vi "PRINT_LABEL.vi"(9 "CURRENT_YEAR_DATA":string, 10 "ECODE 2":string, 11 "connection reference":T1) -> ()   [LabVIEW 2015]
uses:
  <vilib>/addons/database/Connection.llb/Conn ObjectReference.ctl
  Controls/ITEM_INFORMATION_CLUSTER.ctl
  <vilib>/addons/database/_DB Variant To Data/Database Variant To Data.xnode
  <vilib>/addons/database/NI_Database_API.lvlib
  <vilib>/addons/database/Connection.llb/DB Tools Open Connec (String).vi
panel:
  in  "Search button":bool
  in  "Lot Maker":string
  out "Find Array":i32[](array[numeric])
  in  "Location":string
  in  "Maker Code":string
  in  "BUTTON_EXIT":bool
  in  "BUTTON_PRINT":bool
  in  "BUTTON_ADD":bool
  in  "Amount":dbl
  in  "Unit 2":string
  in  "Quantity":dbl
  in  "Lot Size":dbl
  in  "Unit":string
  in  "Item Code (F3)":string
  in  "Part No.(F2)":string
  in  "Barcode (F1)":string
  in  "Offset":dbl
  in  "Length":dbl
  in  "Maker":string(combo)
  in  "Part Name":string(combo)
  in  "Product":string(combo)
  out "ECODE":string
  in  "Invoice Date":timestamp format="%<%d/%m/%Y>T"
  in  "Invoice No.":string
  # "PRINT LABEL"
  # "X"
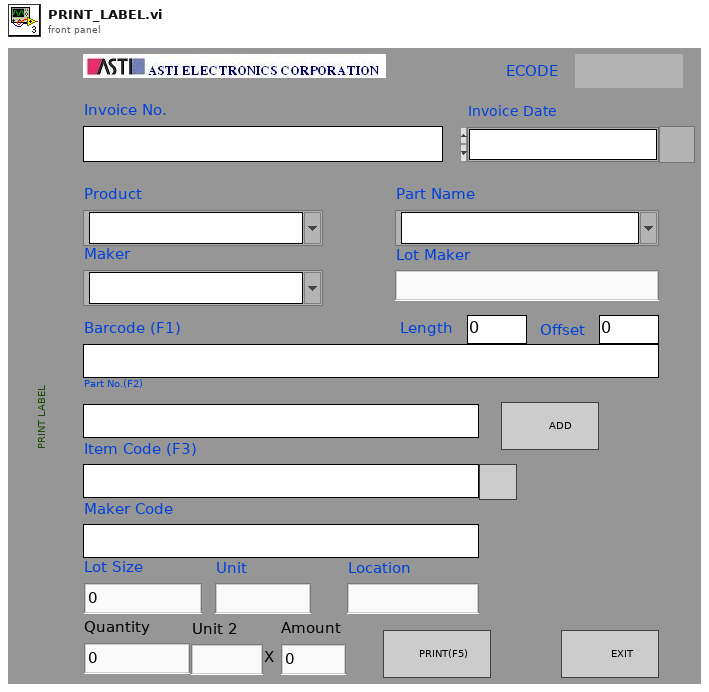
[diagram p1: front panel]
types:
  T1 = typedef "NI_Database_API.lvlib/Conn ObjectReference.ctl" = refnum<k1>
  T2 = typedef "ITEM_INFORMATION_CLUSTER.ctl" = cluster{"PRODUCT":string, "ITEM_CODE":string, "PART_NAME":string, "MAKER":string, "PART_NO":string, "LOT_SIZE":dbl, "UNIT":string, "LENGTH-OFFSET":string, "BARCODE":string, "PROCESS":string, "INVENTORY_LOCAL":string, "TARE":dbl, "SAMPLE":dbl}
  T3 = cluster{"QR_code Text":string, "Lot Maker":string, "Item Code (F3)":string, "date/time string":string, "Invoice No.":string, "Maker":string, "Part No.(F2) ":string, "Location":string, "Product":string, "Qty":string, "ECODE":string}
  T4 = cluster{"PRODUCT":string, "ITEM CODE":string, "PART NAME":string, "MAKER":string, "PART NO":string, "LOT SIZE":dbl, "UNIT":string, "LENGTH-OFFSET":string, "BARCODE":string, "PROCESS":string, "INVENTORY LOCAL":string, "TARE":dbl, "SAMPLE":dbl}
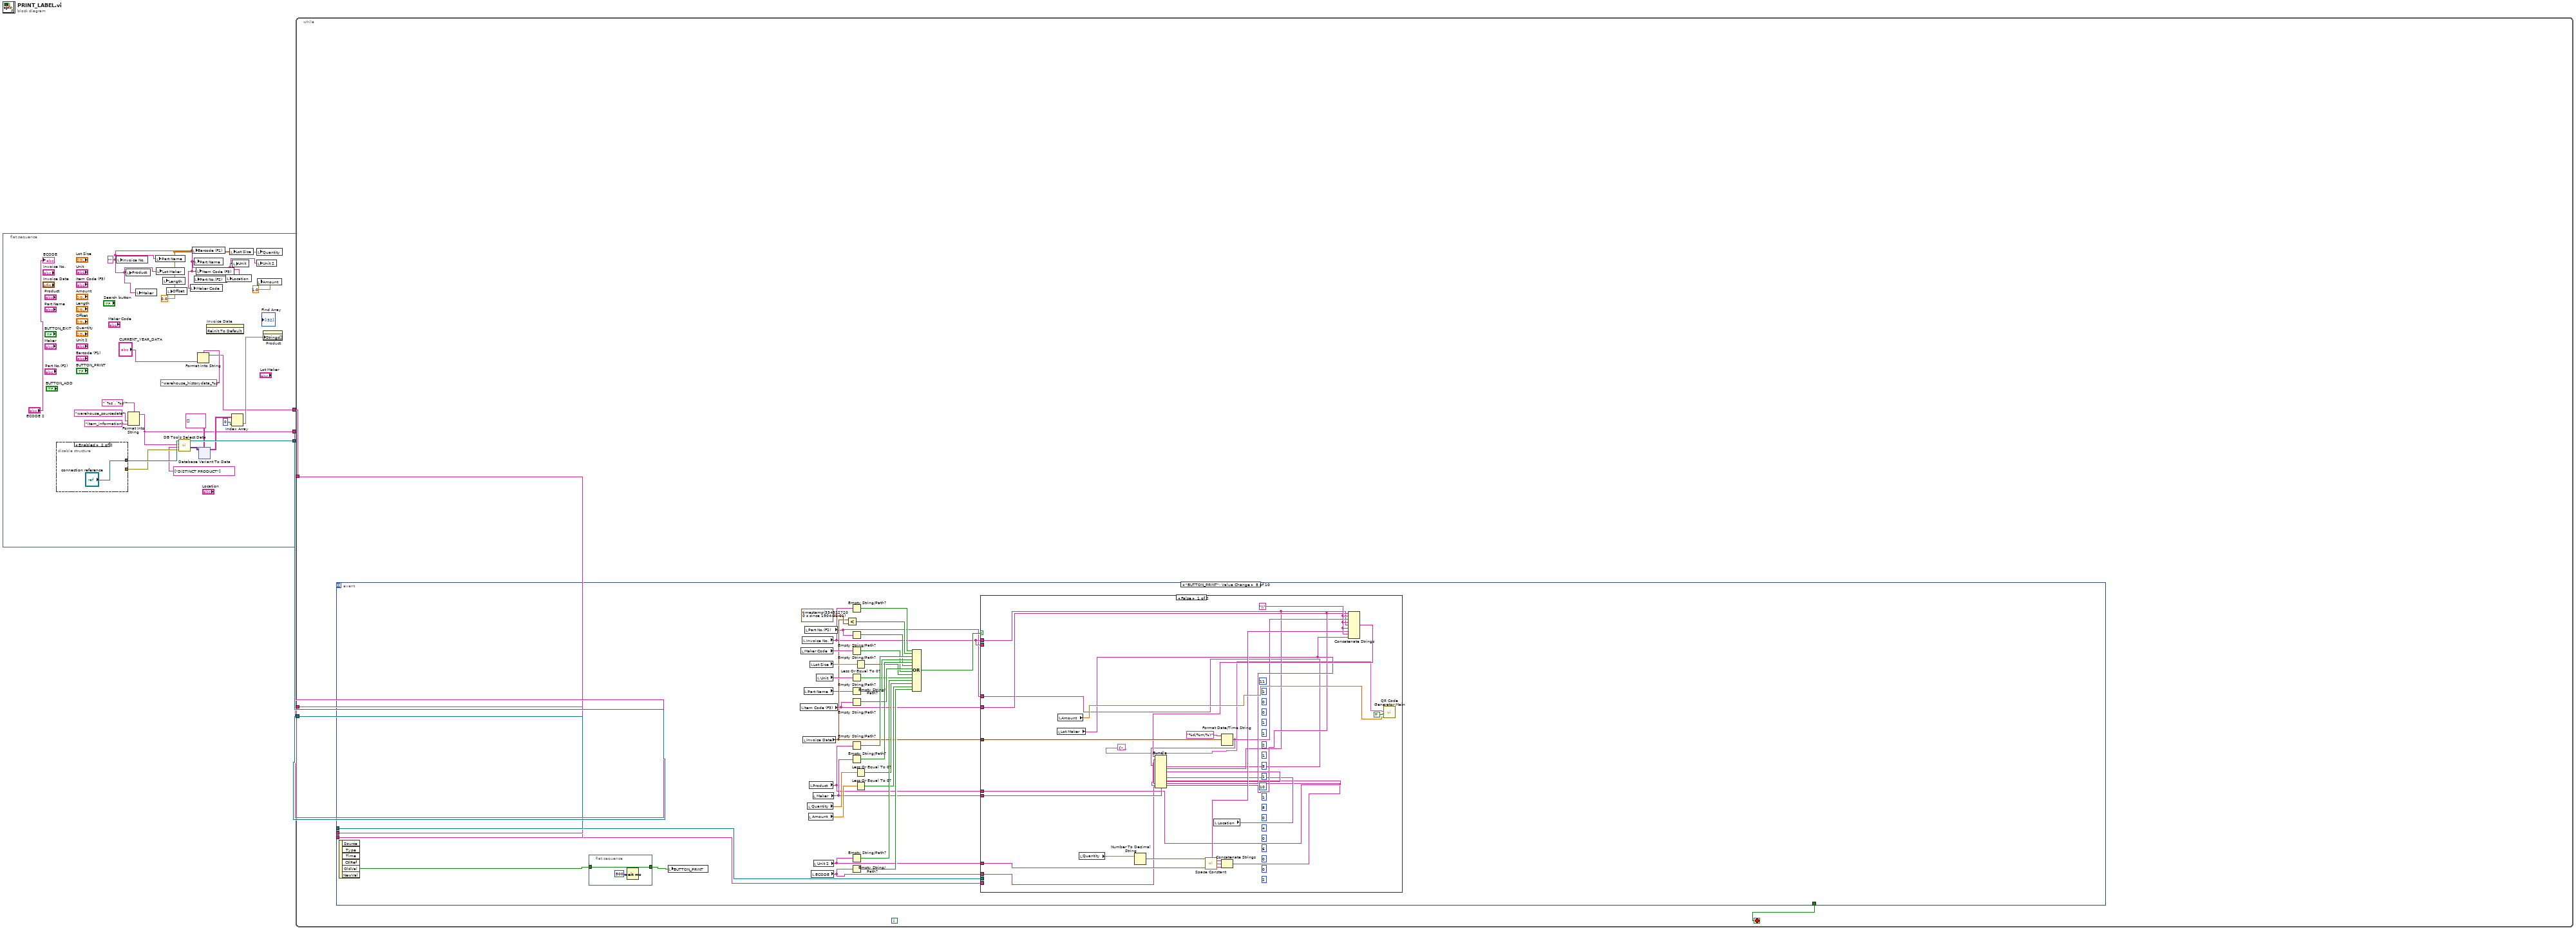
[diagram p0: block diagram]
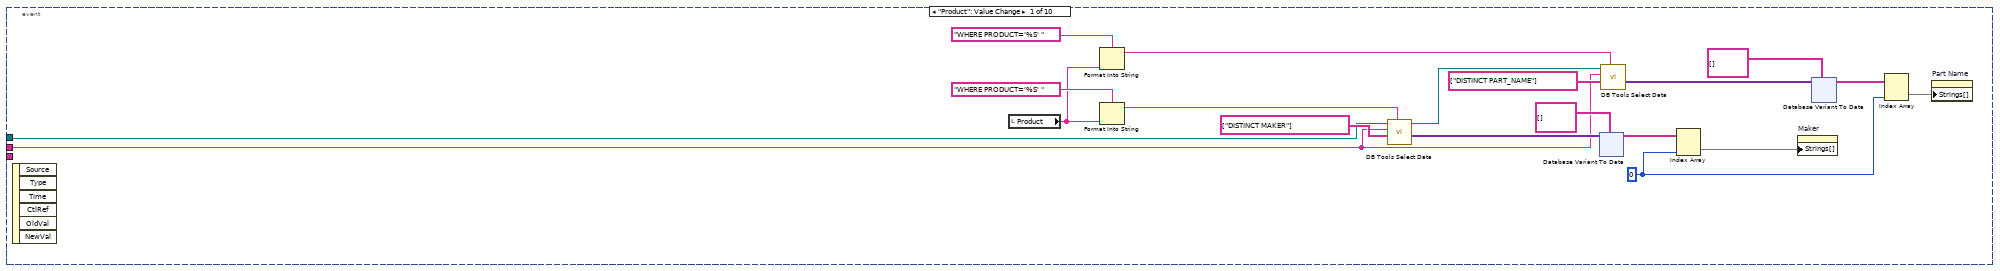
[diagram p2: hidden frame]
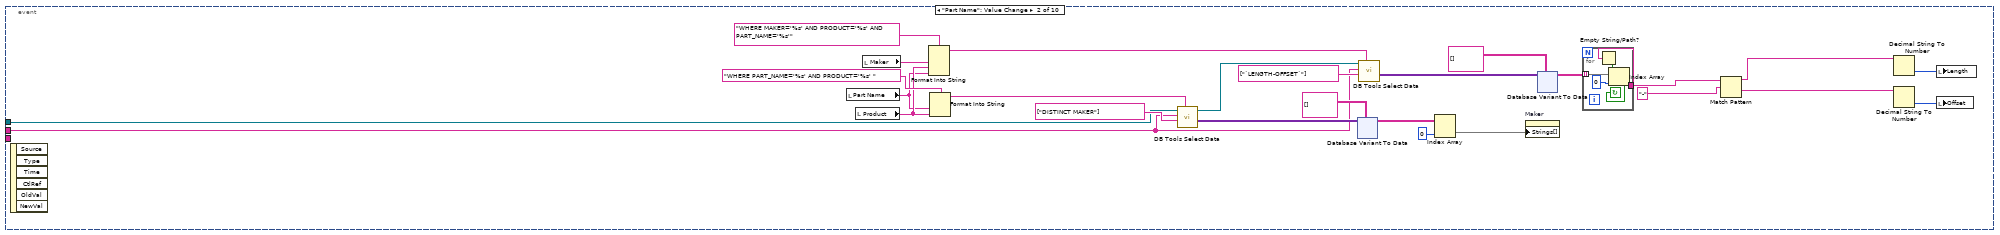
[diagram p3: hidden frame]
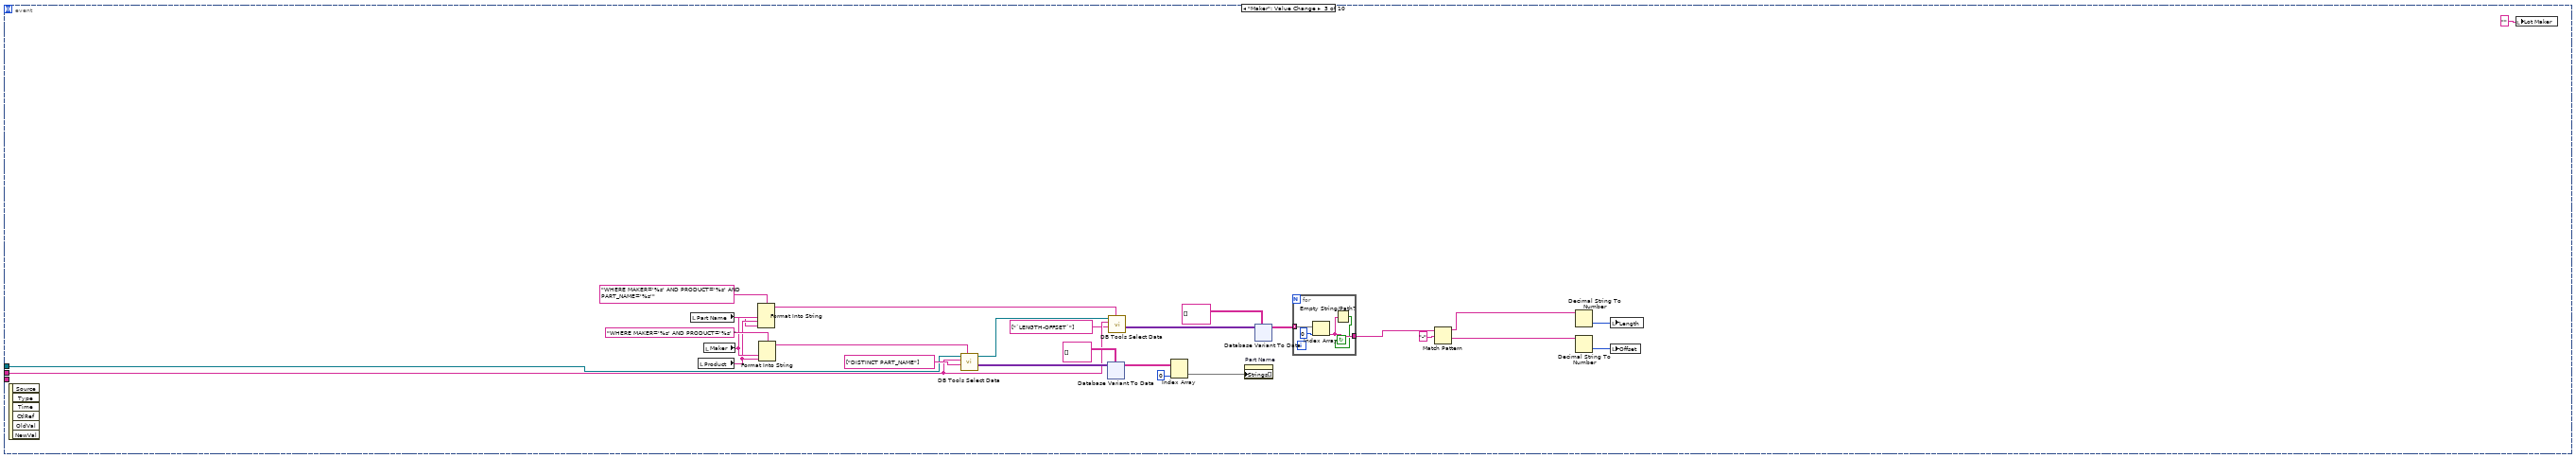
[diagram p4: hidden frame]
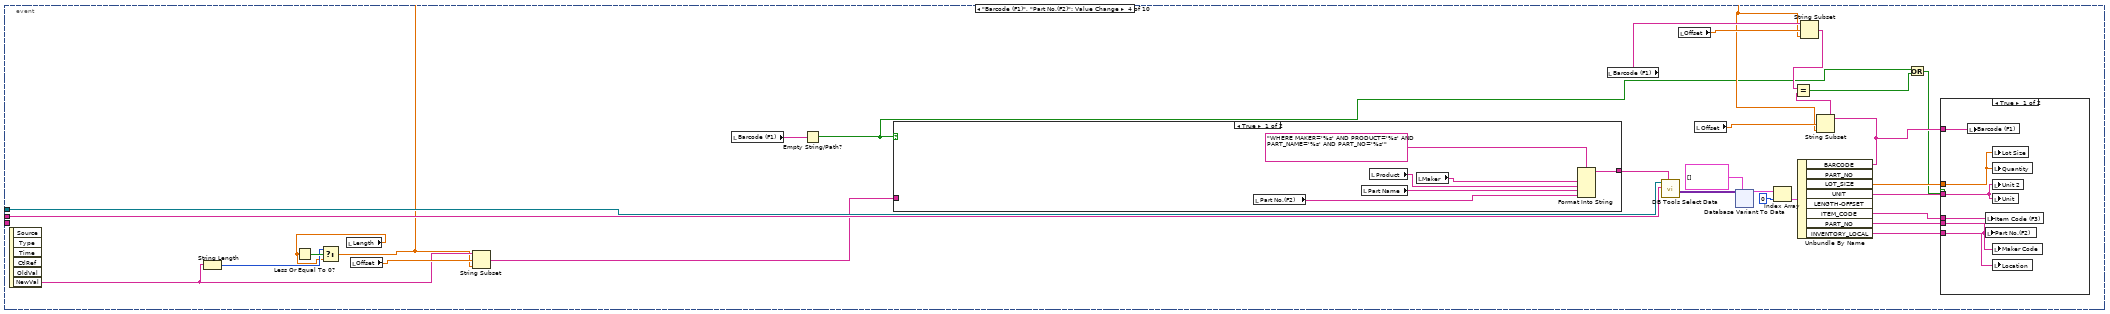
[diagram p5: hidden frame]
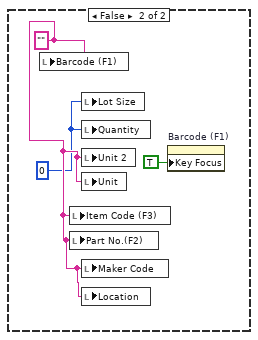
[diagram p6: hidden frame]
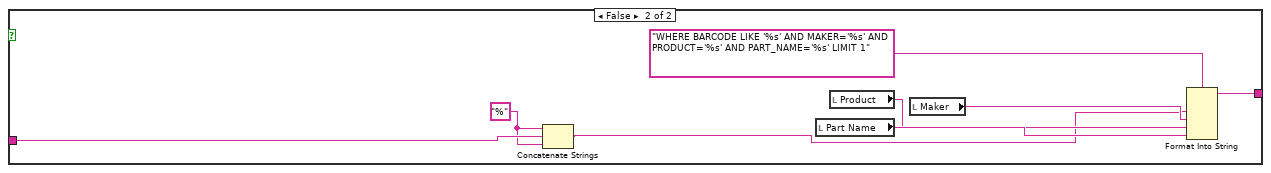
[diagram p7: hidden frame]
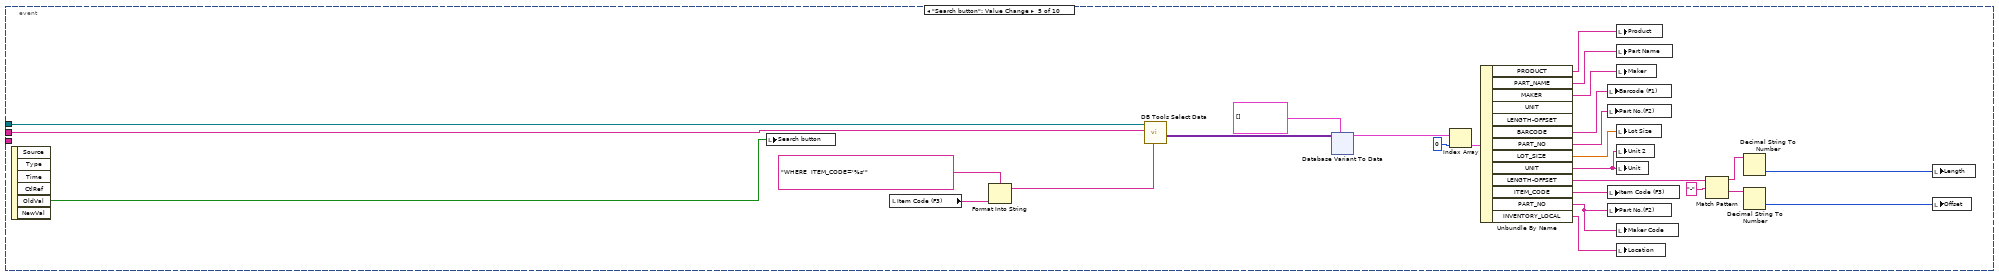
[diagram p8: hidden frame]
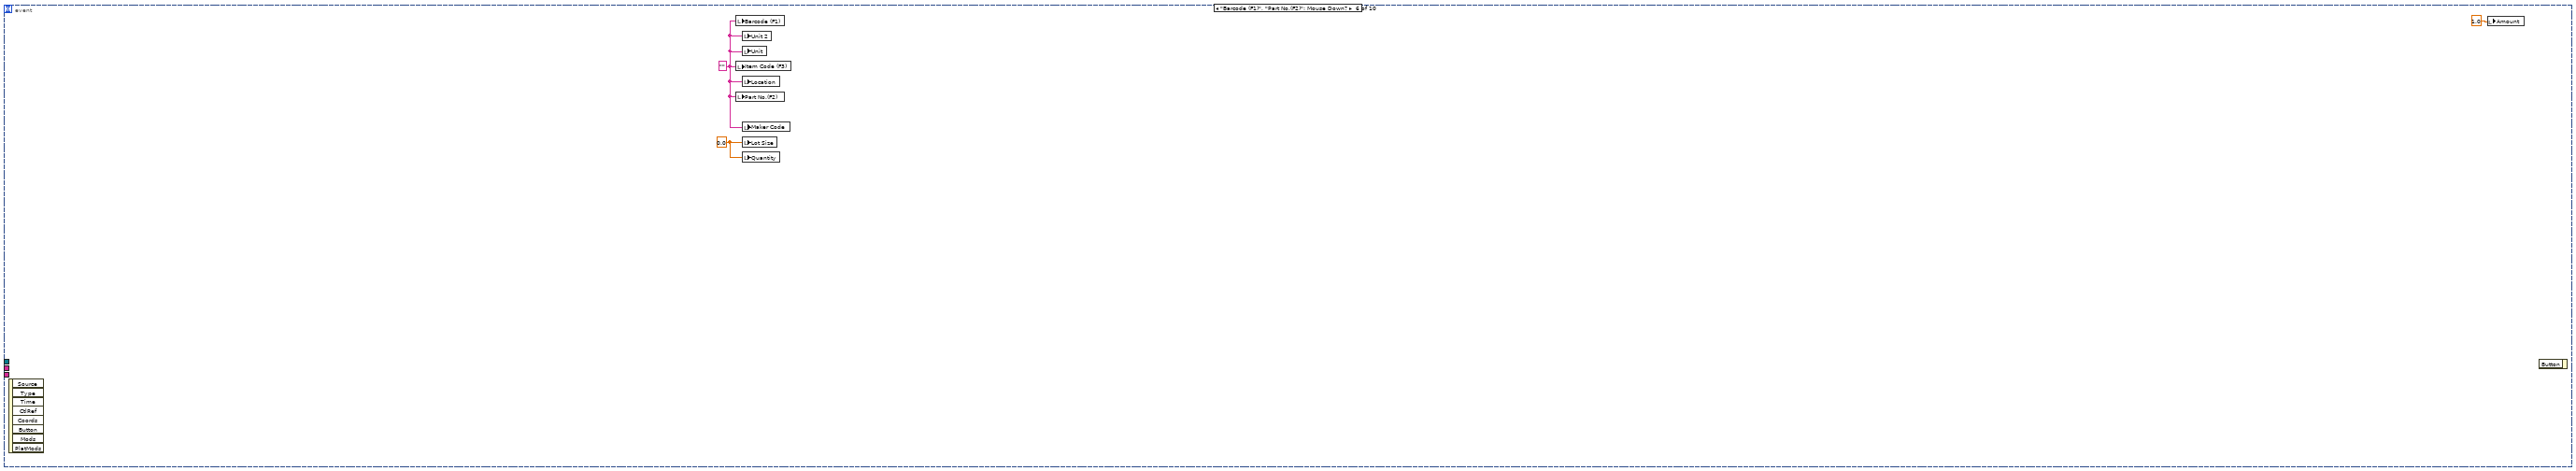
[diagram p9: hidden frame]
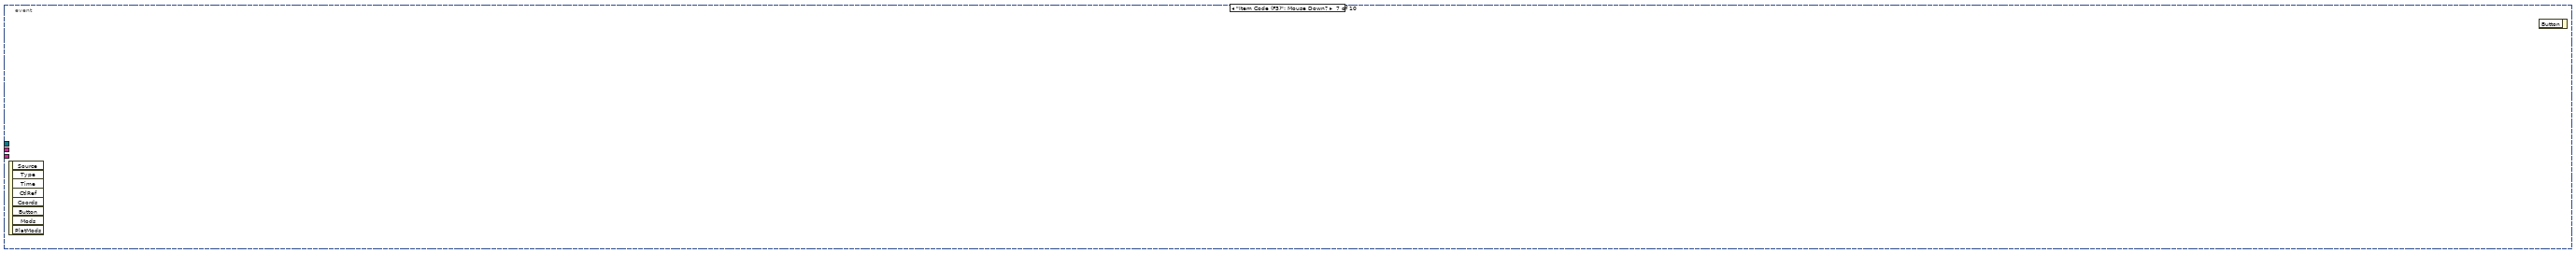
[diagram p10: hidden frame]
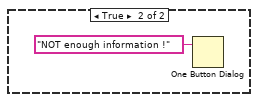
[diagram p11: hidden frame]
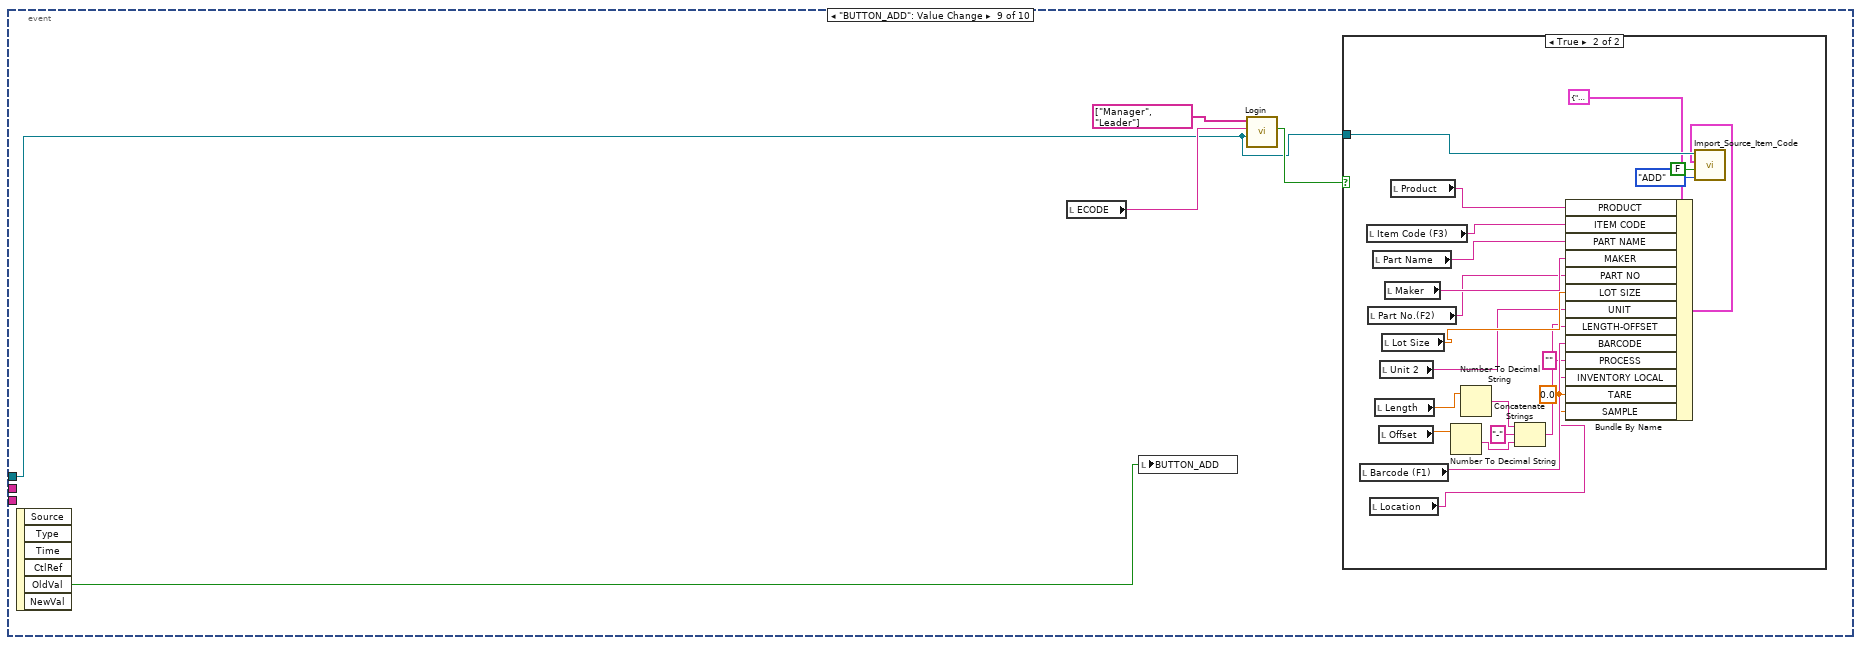
[diagram p12: hidden frame]
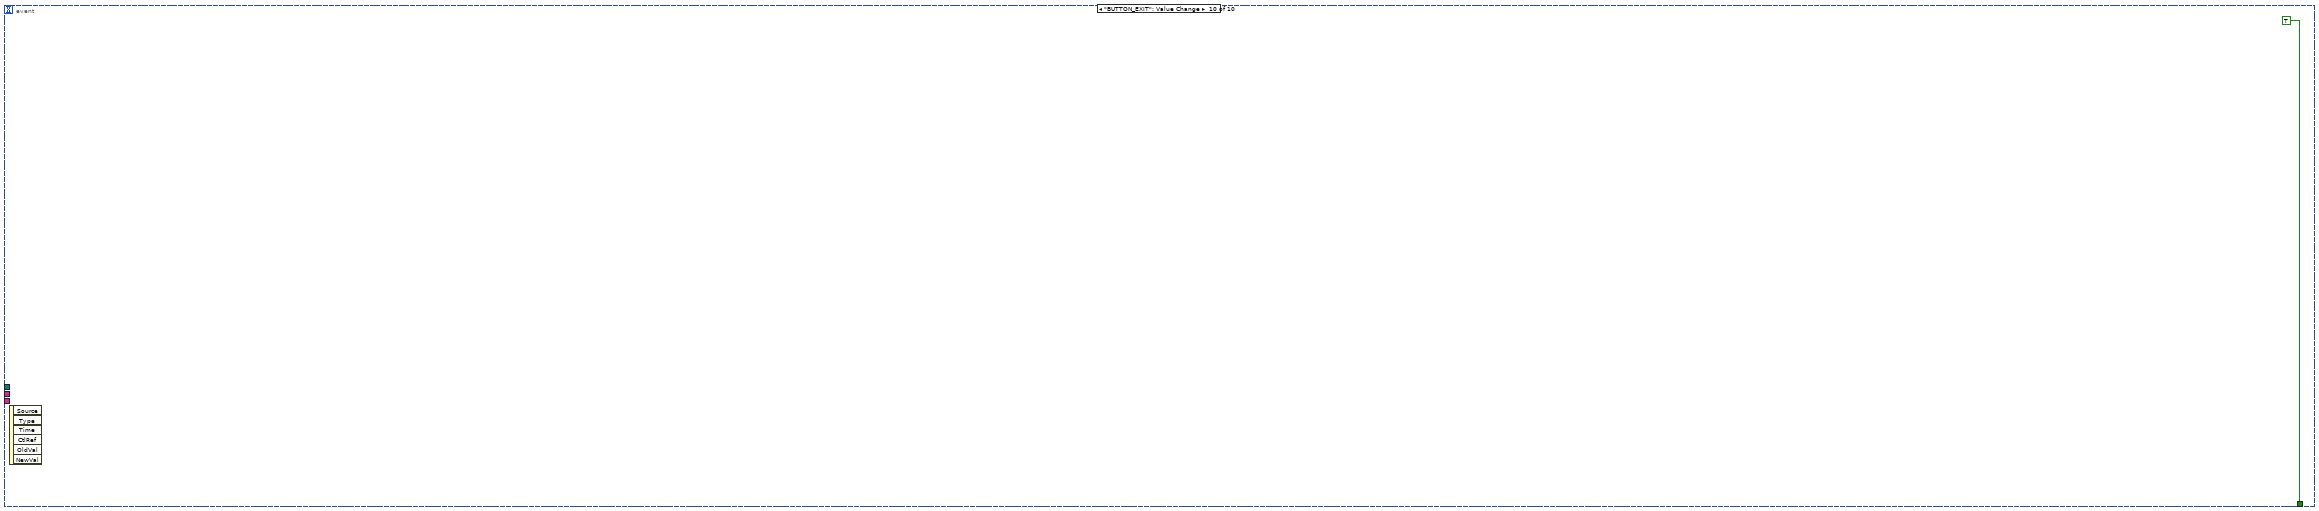
[diagram p14: hidden frame]
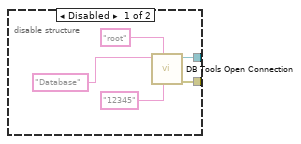
[diagram p15: hidden frame]
diagram:
  n1 = flat-sequence {
    tunnel: [w19] -> w3
    tunnel: [w13] -> w2
    tunnel: [w9] -> w1
    frame #0 {
      w8 = 0.0 ("Length")
      w7 = "" ("Invoice No.")
      n2 = disable-structure shown="Enabled" {
        disable-tunnel: [w25 "connection reference"] -> w21
        disable-tunnel: [w24 _] -> w20
        frame Disabled {
          n3 = call-poly <vilib>:"DB Tools Open Connection.vi"("password"="12345" ("userID"), "userID"="root", "connection information"="Database" ("userID")) -> ("error out"=w24:errorcluster, "connection reference"=w25:T1)  [unwired: 5 in]
        }
        frame Enabled {
        }
      }
      n4 = local write "Invoice No."(w7) -> ()
      n5 = local write "Product"(w7) -> ()
      n6 = Format Into String(format string="`%s`.`%s`" ("table"), "warehouse_sourcedata" ("table"), "item_information" ("table")) -> (resulting string=w13:string)  [unwired: 2 in, 1 out]
      n7 = local write "Maker"(w7) -> ()
      n8 = local write "Part Name"(w7) -> ()
      n9 = local write "Lot Maker"(w7) -> ()
      n10 = local write "Length"(w8) -> ()
      n11 = local write "Offset"(w8) -> ()
      n12 = call <vilib>:"DB Tools Select Data.vi"("error in (no error)"=w20, "columns"=string[] ["DISTINCT PRODUCT"], "table"=w13, "connection reference"=w21) -> ("data"=w18:variant[][], "connection reference out"=w19:T1)  [unwired: 2 in, 1 out]
      n13 = local write "Maker Code"(w7) -> ()
      n14 = local write "Barcode (F1)"(w7) -> ()
      n15 = local write "Part Name"(w7) -> ()
      n16 = local write "Part No.(F2)"(w7) -> ()
      n17 = local write "Item Code (F3)"(w7) -> ()
      n18 = Format Into String(format string="warehouse_historydata_%s" ("table"), "CURRENT_YEAR_DATA") -> (resulting string=w9:string)  [unwired: 2 in, 1 out]
      n19 = xnode "Database Variant To Data"("database variant"=w18, "type"=string[][] []) -> ("data"=w15:string[][])  [unwired: 1 in, 1 out]
      n20 = invoke on="Invoice Date" class="AbsTime (strict)" method="Reinit To Default"() -> ()  [unwired: 3 in, 3 out]
      n21 = local write "Location"(w7) -> ()
      n22 = local write "Lot Size"(w8) -> ()
      n23 = Index Array(array=w15, index (col)=0 ("index (row)")) -> (element=w14:string[])  [unwired: 1 in]
      n24 = local write "Unit"(w7) -> ()
      n25 = local write "Quantity"(w8) -> ()
      n26 = local write "Unit 2"(w7) -> ()
      n27 = local write "Amount"(1.0 ("Amount")) -> ()
      n28 = property on="Product" class="CmbBox"("Strings[]"=w14) -> ()  [unwired: 2 in, 2 out]
      "ECODE" <- "ECODE 2"
    }
  }
  n29 = while {
    tunnel: w3 -> [w76]
    tunnel: w2 -> [w75]
    tunnel: w1 -> [w74]
    stop <- w77 stop-if-true
    n30 = event shown="[7] \"BUTTON_PRINT\": Value Change" {
      selector: _ -> [_ _ _ _ _ _ _ _ _ _]
      dyn-events: _ -> [_ _ _ _ _ _ _ _ _ _]
      timeout: _ -> [_ _ _ _ _ _ _ _ _ _]
      tunnel: [_ _ _ _ _ _ _ _ _ TRUE] -> w77
      tunnel: w76 -> [w92 w203 w322 w449 w912 _ _ w1344 w1390 _]
      tunnel: w75 -> [w79 w188 w318 w448 w911 _ _ _ _ _]
      tunnel: w74 -> [_ _ _ _ _ _ _ w1343 _ _]
      event "Product": Value Change {
        w78 = 0 ("index (row)")
        n31 = event-data() -> ()  [unwired: 1 in, 6 out]
        n32 = local read "Product"() -> (w83:string)
        n33 = Format Into String(format string="WHERE PRODUCT='%S' " ("condition"), w83) -> (resulting string=w89:string)  [unwired: 2 in, 1 out]
        n34 = Format Into String(format string="WHERE PRODUCT='%S' " ("condition"), w83) -> (resulting string=w90:string)  [unwired: 2 in, 1 out]
        n35 = call <vilib>:"DB Tools Select Data.vi"("condition"=w90, "columns"=string[] ["DISTINCT MAKER"], "table"=w79, "connection reference"=w92) -> ("data"=w93:variant[][], "connection reference out"=w82:T1)  [unwired: 2 in, 1 out]
        n36 = xnode "Database Variant To Data"("database variant"=w93, "type"=string[][] []) -> ("data"=w96:string[][])  [unwired: 1 in, 1 out]
        n37 = call <vilib>:"DB Tools Select Data.vi"("condition"=w89, "columns"=string[] ["DISTINCT PART_NAME"], "table"=w79, "connection reference"=w82) -> ("data"=w87:variant[][])  [unwired: 2 in, 2 out]
        n38 = Index Array(array=w96, index (col)=w78) -> (element=w80:string[])  [unwired: 1 in]
        n39 = property on="Maker" class="CmbBox"("Strings[]"=w80) -> ()  [unwired: 2 in, 2 out]
        n40 = xnode "Database Variant To Data"("database variant"=w87, "type"=string[][] []) -> ("data"=w84:string[][])  [unwired: 1 in, 1 out]
        n41 = Index Array(array=w84, index (col)=w78) -> (element=w81:string[])  [unwired: 1 in]
        n42 = property on="Part Name" class="CmbBox"("Strings[]"=w81) -> ()  [unwired: 2 in, 2 out]
      }
      event "Part Name": Value Change {
        n43 = event-data() -> ()  [unwired: 1 in, 6 out]
        n44 = local read "Part Name"() -> (w185:string)
        n45 = local read "Product"() -> (w186:string)
        n46 = local read "Maker"() -> (w187:string)
        n47 = Format Into String(format string="WHERE MAKER='%s' AND PRODUCT='%s' AND PART_NAME='%s'" ("condition"), w187, w186, w185) -> (resulting string=w198:string)  [unwired: 2 in, 1 out]
        n48 = Format Into String(format string="WHERE PART_NAME='%s' AND PRODUCT='%s' " ("condition"), w185, w186) -> (resulting string=w205:string)  [unwired: 2 in, 1 out]
        n49 = call <vilib>:"DB Tools Select Data.vi"("condition"=w205, "columns"=string[] ["DISTINCT MAKER"], "table"=w188, "connection reference"=w203) -> ("data"=w207:variant[][], "connection reference out"=w189:T1)  [unwired: 2 in, 1 out]
        n50 = xnode "Database Variant To Data"("database variant"=w207, "type"=string[][] []) -> ("data"=w210:string[][])  [unwired: 1 in, 1 out]
        n51 = call <vilib>:"DB Tools Select Data.vi"("condition"=w198, "columns"=string[] ["`LENGTH-OFFSET`"], "table"=w188, "connection reference"=w189) -> ("data"=w201:variant[][])  [unwired: 2 in, 2 out]
        n52 = Index Array(array=w210, index (col)=0 ("index (row)")) -> (element=w202:string[])  [unwired: 1 in]
        n53 = property on="Maker" class="CmbBox"("Strings[]"=w202) -> ()  [unwired: 2 in, 2 out]
        n54 = xnode "Database Variant To Data"("database variant"=w201, "type"=string[][] []) -> ("data"=w196:string[][])  [unwired: 1 in, 1 out]
        n55 = for {
          tunnel: w196 -> [w214] mode=indexing
          tunnel: [w212] -> w195
          stop <- w211 continue-if-true
          n56 = Index Array(array=w214, index=0 ("index (row)")) -> (element=w212:string)
          n57 = Empty String/Path?(string/path=w212) -> (empty?=w211:bool)
        }
        n58 = Match Pattern(string=w195, regular expression="-") -> (before substring=w193:string, after substring=w192:string)  [unwired: 1 in, 2 out]
        n59 = Decimal String To Number(string=w193) -> (number=w190:i32)  [unwired: 2 in, 1 out]
        n60 = Decimal String To Number(string=w192) -> (number=w191:i32)  [unwired: 2 in, 1 out]
        n61 = local write "Length"(w190) -> ()
        n62 = local write "Offset"(w191) -> ()
      }
      event "Maker": Value Change {
        n63 = event-data() -> ()  [unwired: 1 in, 6 out]
        n64 = local read "Part Name"() -> (w313:string)
        n65 = local read "Product"() -> (w314:string)
        n66 = local read "Maker"() -> (w315:string)
        n67 = Format Into String(format string="WHERE MAKER='%s' AND PRODUCT='%s' AND PART_NAME='%s'" ("condition"), w315, w314, w313) -> (resulting string=w312:string)  [unwired: 2 in, 1 out]
        n68 = Format Into String(format string="WHERE MAKER='%s' AND PRODUCT='%s' " ("condition"), w315, w314) -> (resulting string=w324:string)  [unwired: 2 in, 1 out]
        n69 = call <vilib>:"DB Tools Select Data.vi"("condition"=w324, "columns"=string[] ["DISTINCT PART_NAME"], "table"=w318, "connection reference"=w322) -> ("data"=w326:variant[][], "connection reference out"=w319:T1)  [unwired: 2 in, 1 out]
        n70 = xnode "Database Variant To Data"("database variant"=w326, "type"=string[][] []) -> ("data"=w329:string[][])  [unwired: 1 in, 1 out]
        n71 = call <vilib>:"DB Tools Select Data.vi"("condition"=w312, "columns"=string[] ["`LENGTH-OFFSET`"], "table"=w318, "connection reference"=w319) -> ("data"=w320:variant[][])  [unwired: 2 in, 2 out]
        n72 = Index Array(array=w329, index (col)=0 ("index (row)")) -> (element=w321:string[])  [unwired: 1 in]
        n73 = property on="Part Name" class="CmbBox"("Strings[]"=w321) -> ()  [unwired: 2 in, 2 out]
        n74 = xnode "Database Variant To Data"("database variant"=w320, "type"=string[][] []) -> ("data"=w310:string[][])  [unwired: 1 in, 1 out]
        n75 = for {
          tunnel: w310 -> [w333] mode=indexing
          tunnel: [w331] -> w309
          stop <- w330 continue-if-true
          n76 = Index Array(array=w333, index=0 ("index (row)")) -> (element=w331:string)
          n77 = Empty String/Path?(string/path=w331) -> (empty?=w330:bool)
        }
        n78 = Match Pattern(string=w309, regular expression="-") -> (before substring=w307:string, after substring=w306:string)  [unwired: 1 in, 2 out]
        n79 = Decimal String To Number(string=w307) -> (number=w304:i32)  [unwired: 2 in, 1 out]
        n80 = Decimal String To Number(string=w306) -> (number=w305:i32)  [unwired: 2 in, 1 out]
        n81 = local write "Length"(w304) -> ()
        n82 = local write "Offset"(w305) -> ()
        n83 = local write "Lot Maker"("" ("Lot Maker")) -> ()
      }
      event "Barcode (F1)", "Part No.(F2)": Value Change {
        n84 = event-data() -> ("NewVal"=w428:string)  [unwired: 1 in, 5 out]
        n85 = String Length(string=w428) -> (length=w427:i32)
        n86 = local read "Length"() -> (w426:dbl)
        n87 = Less Or Equal To 0?(x=w426) -> (x <= 0?=w429:bool)
        n88 = Select(t=w427, s=w429, f=w426) -> (s? t:f=w425:dbl)
        n89 = local read "Offset"() -> (w437:dbl)
        n90 = String Subset(string=w428, offset (0)=w437, length (rest)=w425) -> (substring=w436:string)
        n91 = local read "Barcode (F1)"() -> (w439:string)
        n92 = Empty String/Path?(string/path=w439) -> (empty?=w423:bool)
        n93 = case shown="True" w423 {
          tunnel: [w464 w472] -> w450
          tunnel: w436 -> [_ w470]
          frame True {
            n94 = local read "Part No.(F2)"() -> (w461:string)
            n95 = local read "Part Name"() -> (w465:string)
            n96 = local read "Product"() -> (w462:string)
            n97 = local read "Maker"() -> (w463:string)
            n98 = Format Into String(format string="WHERE MAKER='%s' AND PRODUCT='%s' AND PART_NAME='%s' AND PART_NO='%s'" ("condition"), w463, w462, w465, w461) -> (resulting string=w464:string)  [unwired: 2 in, 1 out]
          }
          frame False {
            w469 = "%"
            n99 = Concatenate Strings(w469, w470, w469) -> (w467:string)
            n100 = local read "Part Name"() -> (w473:string)
            n101 = local read "Product"() -> (w471:string)
            n102 = local read "Maker"() -> (w468:string)
            n103 = Format Into String(format string="WHERE BARCODE LIKE '%s' AND MAKER='%s' AND PRODUCT='%s' AND PART_NAME='%s' LIMIT 1" ("condition"), w467, w468, w471, w473) -> (resulting string=w472:string)  [unwired: 2 in, 1 out]
          }
        }
        n104 = local read "Barcode (F1)"() -> (w432:string)
        n105 = call <vilib>:"DB Tools Select Data.vi"("condition"=w450, "table"=w448, "connection reference"=w449) -> ("data"=w451:variant[][])  [unwired: 3 in, 2 out]
        n106 = local read "Offset"() -> (w433:dbl)
        n107 = local read "Offset"() -> (w435:dbl)
        n108 = xnode "Database Variant To Data"("database variant"=w451, "type"=T2[] []) -> ("data"=w446:T2[])  [unwired: 1 in, 1 out]
        n109 = Index Array(array=w446, index=0) -> (element=w444:T2)
        n110 = Unbundle By Name(w444) -> ("BARCODE"=w430:string, "LOT_SIZE"=w443:dbl, "UNIT"=w442:string, "ITEM_CODE"=w438:string, "PART_NO"=w441:string, "INVENTORY_LOCAL"=w440:string)  [unwired: 2 out]
        n111 = String Subset(string=w432, offset (0)=w433, length (rest)=w425) -> (substring=w431:string)
        n112 = String Subset(string=w430, offset (0)=w435, length (rest)=w425) -> (substring=w434:string)
        n113 = Equal?(x=w431, y=w434) -> (x = y?=w424:bool)
        n114 = Or(x=w423, y=w424) -> (x .or. y?=w422:bool)
        n115 = case shown="True" w422 {
          tunnel: w443 -> [w457 _]
          tunnel: w442 -> [w456 _]
          tunnel: w441 -> [w455 _]
          tunnel: w440 -> [w454 _]
          tunnel: w438 -> [w453 _]
          tunnel: w430 -> [w452 _]
          frame True {
            n116 = local write "Barcode (F1)"(w452) -> ()
            n117 = local write "Item Code (F3)"(w453) -> ()
            n118 = local write "Part No.(F2)"(w455) -> ()
            n119 = local write "Lot Size"(w457) -> ()
            n120 = local write "Quantity"(w457) -> ()
            n121 = local write "Unit 2"(w456) -> ()
            n122 = local write "Unit"(w456) -> ()
            n123 = local write "Maker Code"(w455) -> ()
            n124 = local write "Location"(w454) -> ()
          }
          frame False {
            w459 = 0
            w460 = ""
            n125 = local write "Barcode (F1)"(w460) -> ()
            n126 = local write "Item Code (F3)"(w460) -> ()
            n127 = local write "Part No.(F2)"(w460) -> ()
            n128 = local write "Lot Size"(w459) -> ()
            n129 = local write "Quantity"(w459) -> ()
            n130 = local write "Unit 2"(w460) -> ()
            n131 = local write "Unit"(w460) -> ()
            n132 = local write "Maker Code"(w460) -> ()
            n133 = local write "Location"(w460) -> ()
            n134 = property on="Barcode (F1)" class="Str"("Key Focus"=TRUE) -> ()  [unwired: 2 in, 2 out]
          }
        }
      }
      event "Search button": Value Change {
        n135 = event-data() -> ("OldVal"=w888:bool)  [unwired: 1 in, 5 out]
        n136 = local write "Search button"(w888) -> ()
        n137 = local read "Item Code (F3)"() -> (w893:string)
        n138 = Format Into String(format string="WHERE  ITEM_CODE='%s'" ("condition"), w893) -> (resulting string=w913:string)  [unwired: 2 in, 1 out]
        n139 = call <vilib>:"DB Tools Select Data.vi"("condition"=w913, "table"=w911, "connection reference"=w912) -> ("data"=w914:variant[][])  [unwired: 3 in, 2 out]
        n140 = xnode "Database Variant To Data"("database variant"=w914, "type"=T2[] []) -> ("data"=w909:T2[])  [unwired: 1 in, 1 out]
        n141 = Index Array(array=w909, index=0) -> (element=w907:T2)
        n142 = Unbundle By Name(w907) -> ("PRODUCT"=w891:string, "PART_NAME"=w890:string, "MAKER"=w889:string, "BARCODE"=w900:string, "PART_NO"=w906:string, "LOT_SIZE"=w904:dbl, "UNIT"=w903:string, "LENGTH-OFFSET"=w905:string, "ITEM_CODE"=w899:string, "PART_NO"=w902:string, "INVENTORY_LOCAL"=w901:string)  [unwired: 2 out]
        n143 = local write "Barcode (F1)"(w900) -> ()
        n144 = local write "Part No.(F2)"(w906) -> ()
        n145 = local write "Item Code (F3)"(w899) -> ()
        n146 = local write "Part No.(F2)"(w902) -> ()
        n147 = local write "Product"(w891) -> ()
        n148 = local write "Part Name"(w890) -> ()
        n149 = local write "Maker"(w889) -> ()
        n150 = local write "Lot Size"(w904) -> ()
        n151 = local write "Unit 2"(w903) -> ()
        n152 = local write "Unit"(w903) -> ()
        n153 = local write "Maker Code"(w902) -> ()
        n154 = local write "Location"(w901) -> ()
        n155 = Match Pattern(string=w905, regular expression="-") -> (before substring=w897:string, after substring=w896:string)  [unwired: 1 in, 2 out]
        n156 = Decimal String To Number(string=w897) -> (number=w894:i32)  [unwired: 2 in, 1 out]
        n157 = Decimal String To Number(string=w896) -> (number=w895:i32)  [unwired: 2 in, 1 out]
        n158 = local write "Length"(w894) -> ()
        n159 = local write "Offset"(w895) -> ()
      }
      event "Barcode (F1)", "Part No.(F2)": Mouse Down? {
        w1328 = 0.0 ("Length")
        w1329 = "" ("Invoice No.")
        n160 = event-data() -> ()  [unwired: 1 in, 8 out]
        n161 = local write "Barcode (F1)"(w1329) -> ()
        n162 = local write "Item Code (F3)"(w1329) -> ()
        n163 = local write "Part No.(F2)"(w1329) -> ()
        n164 = local write "Unit 2"(w1329) -> ()
        n165 = local write "Unit"(w1329) -> ()
        n166 = local write "Location"(w1329) -> ()
        n167 = local write "Maker Code"(w1329) -> ()
        n168 = local write "Lot Size"(w1328) -> ()
        n169 = local write "Quantity"(w1328) -> ()
        n170 = local write "Amount"(1.0 ("Amount")) -> ()
        n171 = event-data() -> ()  [unwired: 2 in, 1 out]
      }
      event "Item Code (F3)": Mouse Down? {
        n172 = event-data() -> ()  [unwired: 1 in, 8 out]
        n173 = event-data() -> ()  [unwired: 2 in, 1 out]
      }
      event "BUTTON_PRINT": Value Change {
        n174 = event-data() -> ("OldVal"=w1332:bool)  [unwired: 1 in, 5 out]
        n175 = flat-sequence {
          tunnel: [w1366] -> w1331
          tunnel: w1332 -> [w1366]
          frame #0 {
            n176 = Wait (ms)(milliseconds to wait=u32 500) -> ()  [unwired: 1 out]
          }
        }
        n177 = local write "BUTTON_PRINT"(w1331) -> ()
        n178 = local read "Item Code (F3)"() -> (w1341:string)
        n179 = local read "Maker Code"() -> (w1363:string)
        n180 = local read "Invoice No."() -> (w1339:string)
        n181 = local read "Invoice Date"() -> (w1340:timestamp)
        n182 = local read "Part Name"() -> (w1338:string)
        n183 = local read "Part No.(F2)"() -> (w1334:string)
        n184 = local read "Quantity"() -> (w1360:dbl)
        n185 = local read "Amount"() -> (w1359:dbl)
        n186 = local read "Product"() -> (w1336:string)
        n187 = local read "Lot Size"() -> (w1362:dbl)
        n188 = local read "ECODE"() -> (w1333:string)
        n189 = local read "Maker"() -> (w1337:string)
        n190 = local read "Unit 2"() -> (w1335:string)
        n191 = local read "Unit"() -> (w1361:string)
        n192 = Less?(x=w1340, y=timestamp(3345127200 s since 1904-01-01)) -> (x < y?=w1357:bool)
        n193 = Empty String/Path?(string/path=w1339) -> (empty?=w1358:bool)
        n194 = Empty String/Path?(string/path=w1334) -> (empty?=w1353:bool)
        n195 = Empty String/Path?(string/path=w1363) -> (empty?=w1351:bool)
        n196 = Empty String/Path?(string/path=w1361) -> (empty?=w1349:bool)
        n197 = Empty String/Path?(string/path=w1338) -> (empty?=w1355:bool)
        n198 = Empty String/Path?(string/path=w1341) -> (empty?=w1352:bool)
        n199 = Empty String/Path?(string/path=w1336) -> (empty?=w1356:bool)
        n200 = Empty String/Path?(string/path=w1337) -> (empty?=w1354:bool)
        n201 = Empty String/Path?(string/path=w1335) -> (empty?=w1348:bool)
        n202 = Empty String/Path?(string/path=w1333) -> (empty?=w1342:bool)
        n203 = Less Or Equal To 0?(x=w1362) -> (x <= 0?=w1350:bool)
        n204 = Less Or Equal To 0?(x=w1360) -> (x <= 0?=w1347:bool)
        n205 = Less Or Equal To 0?(x=w1359) -> (x <= 0?=w1346:bool)
        n206 = Compound Arithmetic op=OR(w1358, w1357, w1356, w1355, w1354, w1353, w1352, w1351, w1350, w1349, w1348, w1347, w1346, w1342) -> (w1345:bool)
        n207 = case shown="False" w1345 {
          tunnel: w1344 -> [_ _]
          tunnel: w1343 -> [_ _]
          tunnel: w1339 -> [_ _]
          tunnel: w1341 -> [w1377 _]
          tunnel: w1340 -> [w1388 _]
          tunnel: w1339 -> [w1375 _]
          tunnel: w1334 -> [w1373 _]
          tunnel: w1337 -> [w1374 _]
          tunnel: w1336 -> [w1371 _]
          tunnel: w1333 -> [w1369 _]
          tunnel: w1335 -> [w1383 _]
          frame False {
            (unwired) 2 ("disabled index (col)")
            (unwired) 0 ("index (row)")
            (unwired) 0 ("disabled index (col)")
            (unwired) 6 ("index (row)")
            (unwired) 0 ("disabled index (col)")
            (unwired) 4 ("index (row)")
            (unwired) 0 ("disabled index (col)")
            (unwired) 8 ("index (row)")
            (unwired) 1 ("disabled index (col)")
            (unwired) 10 ("index (row)")
            (unwired) 1 ("disabled index (col)")
            (unwired) 9 ("index (row)")
            (unwired) 1 ("disabled index (col)")
            (unwired) 2 ("index (row)")
            (unwired) 1 ("disabled index (col)")
            (unwired) 1 ("index (row)")
            (unwired) 0 ("disabled index (col)")
            (unwired) 0 ("index (row)")
            (unwired) 1 ("disabled index (col)")
            (unwired) 11 ("index (row)")
            w1381 = "\\" ("string")
            n208 = local read "Lot Maker"() -> (w1378:string)
            n209 = local read "Amount"() -> (w1382:dbl)
            n210 = local read "Quantity"() -> (w1385:dbl)
            n211 = Number To Decimal String(number=w1385) -> (decimal integer string=w1380:string)  [unwired: 1 in]
            n212 = call <vilib>:"Space Constant.vi"() -> ("String"=w1384:string)
            n213 = local read "Location"() -> (w1372:string)
            n214 = Concatenate Strings(w1380, w1384, w1383) -> (w1370:string)
            n215 = Format Date/Time String(time format string (%c)="%d/%m/%Y", seconds (now)=w1388) -> (date/time string=w1376:string)  [unwired: 1 in]
            n216 = Concatenate Strings(w1377, w1381, w1376, w1381, w1375, w1381, w1380, w1381, w1378) -> (w1379:string)
            n217 = Bundle(cluster=T3 {"QR_code Text"="", "Lot Maker"="", "Item Code (F3)"="", "date/time string"="", "Invoice No."="", "Maker"="", "Part No.(F2) "="", "Location"="", "Product"="", "Qty"="", "ECODE"=""} ("output cluster"), "QR_code Text"=w1379, "Lot Maker"=w1378, "Item Code (F3)"=w1377, "date/time string"=w1376, "Invoice No."=w1375, "Maker"=w1374, "Part No.(F2)"=w1373, "Location"=w1372, "Product"=w1371, "Qty"=w1370, "ECODE"=w1369) -> (w1367:T3)
            n218 = call "QR Code Generator Main.vi"("number of copies (1)"=w1382, "Print Button"=TRUE, "output cluster"=w1367) -> ()  [unwired: 9 in]
          }
          frame True {
            n219 = One Button Dialog(message="NOT enough information !") -> ()  [unwired: 1 in, 1 out]
          }
        }
      }
      event "BUTTON_ADD": Value Change {
        n220 = event-data() -> ("OldVal"=w1394:bool)  [unwired: 1 in, 5 out]
        n221 = local read "ECODE"() -> (w1393:string)
        n222 = local write "BUTTON_ADD"(w1394) -> ()
        n223 = call "Login.vi"("connection reference"=w1390, "ACCOUNT:"=w1393, "Permission"=string[] ["Manager", "Leader"]) -> ("OK"=w1392:bool)  [unwired: 7 in, 1 out]
        n224 = case shown="True" w1392 {
          tunnel: w1390 -> [_ w1416]
          frame False {
          }
          frame True {
            w1398 = 0.0 ("TARE")
            n225 = local read "Barcode (F1)"() -> (w1401:string)
            n226 = local read "Item Code (F3)"() -> (w1413:string)
            n227 = local read "Part No.(F2)"() -> (w1410:string)
            n228 = local read "Location"() -> (w1400:string)
            n229 = local read "Part Name"() -> (w1412:string)
            n230 = local read "Length"() -> (w1406:dbl)
            n231 = local read "Offset"() -> (w1407:dbl)
            n232 = local read "Unit 2"() -> (w1408:string)
            n233 = local read "Lot Size"() -> (w1409:dbl)
            n234 = local read "Maker"() -> (w1411:string)
            n235 = local read "Product"() -> (w1414:string)
            n236 = Number To Decimal String(number=w1407) -> (decimal integer string=w1403:string)  [unwired: 1 in]
            n237 = Number To Decimal String(number=w1406) -> (decimal integer string=w1404:string)  [unwired: 1 in]
            n238 = Concatenate Strings(w1404, "-" ("string"), w1403) -> (w1402:string)
            n239 = Bundle By Name(cluster=T4 {"PRODUCT"="", "ITEM CODE"="", "PART NAME"="", "MAKER"="", "PART NO"="", "LOT SIZE"=0.0, "UNIT"="", "LENGTH-OFFSET"="", "BARCODE"="", "PROCESS"="", "INVENTORY LOCAL"="", "TARE"=0.0, "SAMPLE"=0.0} ("ITEM_DATA"), "PRODUCT"=w1414, "ITEM CODE"=w1413, "PART NAME"=w1412, "MAKER"=w1411, "PART NO"=w1410, "LOT SIZE"=w1409, "UNIT"=w1408, "LENGTH-OFFSET"=w1402, "BARCODE"=w1401, "PROCESS"="", "INVENTORY LOCAL"=w1400, "TARE"=w1398, "SAMPLE"=w1398) -> (w1395:T4)
            n240 = call "Import_Source_Item_Code.vi"("CONTROL Control"=enum32{"IMPRORT", "ADD"}."ADD", "UPDATE ONLY"=FALSE, "ITEM_DATA"=w1395, "connection reference"=w1416) -> ()  [unwired: 8 in]
          }
        }
      }
      event "BUTTON_EXIT": Value Change {
        n241 = event-data() -> ()  [unwired: 1 in, 6 out]
      }
    }
  }
